vi "Do Nothing subVI test.vi"(10 "String":string) -> (2 "String 2":string)   [LabVIEW 2020]
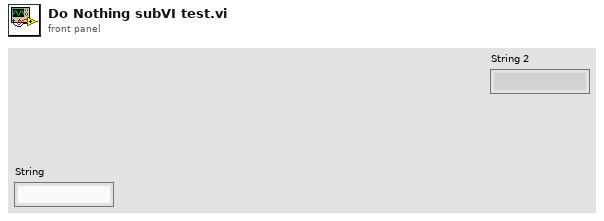
[diagram p1: front panel]
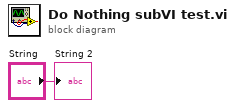
[diagram p0: block diagram]
diagram:
  "String 2" <- "String"
